vi "Gather Input.vi"(4 "Shifter":T1, 7 "Gamepad":T1, 8 "Joystick Right":T1, 11 "Joystick Left":T1) -> ()   [LabVIEW 2016]
uses:
  <vilib>/Rock Robotics/WPI/Joystick/WPI_JoystickDevRef.ctl
  <vilib>/Rock Robotics/WPI/Joystick/WPI_JoystickDeviceEnum.ctl
  Joystick Values.vi
panel:
  in  "Gamepad 2":T1
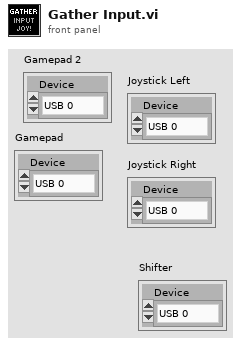
[diagram p1: front panel]
types:
  T1 = typedef "WPI_JoystickDevRef.ctl" = cluster{"Device":T2}
  T2 = typedef "WPI_JoystickDeviceEnum.ctl" = enum16{"USB 0", "USB 1", "USB 2", "USB 3", "USB 4", "USB 5"}
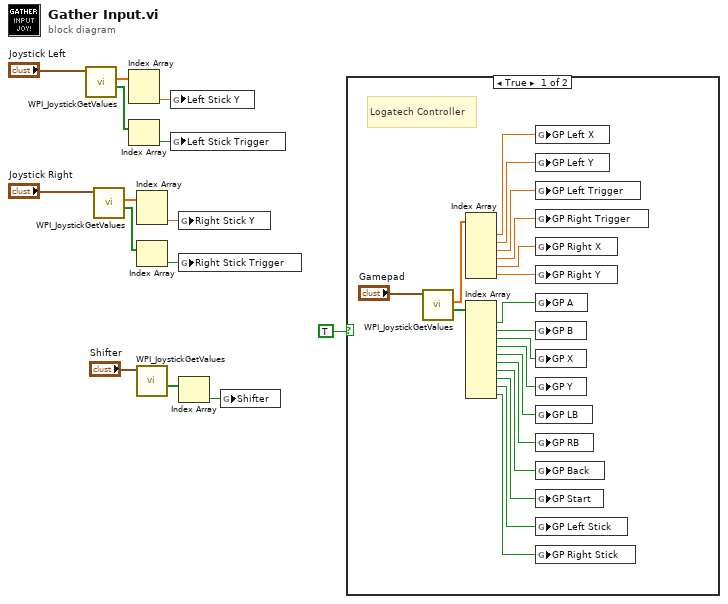
[diagram p0: block diagram]
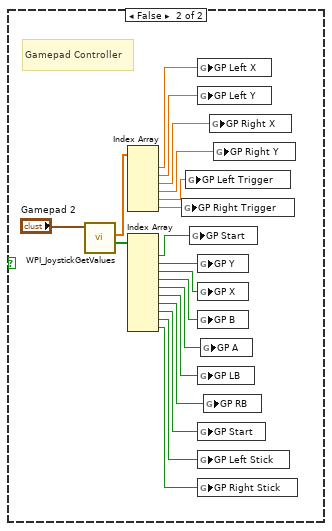
[diagram p2: hidden frame]
diagram:
  n1 = call <vilib>:"WPI_JoystickGetValues.vi"("JoystickDevRef"="Joystick Left") -> ("Buttons"=w6:bool[], "Axes"=w5:dbl[])  [unwired: 6 in, 3 out]
  n2 = call <vilib>:"WPI_JoystickGetValues.vi"("JoystickDevRef"="Joystick Right") -> ("Buttons"=w12:bool[], "Axes"=w10:dbl[])  [unwired: 6 in, 3 out]
  n3 = Index Array(array=w5) -> (element #2=w7:dbl)  [unwired: 2 in, 1 out]
  n4 = Index Array(array=w6) -> (element=w8:bool)  [unwired: 1 in]
  n5 = Index Array(array=w10) -> (element #2=w9:dbl)  [unwired: 2 in, 1 out]
  n6 = Index Array(array=w12) -> (element=w11:bool)  [unwired: 1 in]
  n7 = call <vilib>:"WPI_JoystickGetValues.vi"("JoystickDevRef"="Shifter") -> ("Buttons"=w3:bool[])  [unwired: 6 in, 4 out]
  n8 = global write "Joystick Values.vi" "Left Stick Y"(w7) -> ()
  n9 = global write "Joystick Values.vi" "Left Stick Trigger"(w8) -> ()
  n10 = global write "Joystick Values.vi" "Right Stick Y"(w9) -> ()
  n11 = global write "Joystick Values.vi" "Right Stick Trigger"(w11) -> ()
  n12 = Index Array(array=w3) -> (element=w2:bool)  [unwired: 1 in]
  n13 = global write "Joystick Values.vi" "Shifter"(w2) -> ()
  n14 = case shown="True" TRUE {
    frame True {
      # "Logatech Controller"
      n15 = call <vilib>:"WPI_JoystickGetValues.vi"("JoystickDevRef"="Gamepad") -> ("Buttons"=w32:bool[], "Axes"=w20:dbl[])  [unwired: 6 in, 3 out]
      n16 = Index Array(array=w20) -> (element #1=w21:dbl, element #2=w19:dbl, element #3=w16:dbl, element #4=w15:dbl, element #5=w18:dbl, element #6=w17:dbl)  [unwired: 6 in]
      n17 = Index Array(array=w32) -> (element #1=w31:bool, element #2=w30:bool, element #3=w29:bool, element #4=w28:bool, element #5=w27:bool, element #6=w26:bool, element #7=w25:bool, element #8=w24:bool, element #9=w23:bool, element #10=w22:bool)  [unwired: 10 in]
      n18 = global write "Joystick Values.vi" "GP Left X"(w21) -> ()
      n19 = global write "Joystick Values.vi" "GP Left Y"(w19) -> ()
      n20 = global write "Joystick Values.vi" "GP Left Trigger"(w16) -> ()
      n21 = global write "Joystick Values.vi" "GP Right Trigger"(w15) -> ()
      n22 = global write "Joystick Values.vi" "GP Right X"(w18) -> ()
      n23 = global write "Joystick Values.vi" "GP Right Y"(w17) -> ()
      n24 = global write "Joystick Values.vi" "GP A"(w31) -> ()
      n25 = global write "Joystick Values.vi" "GP B"(w30) -> ()
      n26 = global write "Joystick Values.vi" "GP X"(w29) -> ()
      n27 = global write "Joystick Values.vi" "GP Y"(w28) -> ()
      n28 = global write "Joystick Values.vi" "GP LB"(w27) -> ()
      n29 = global write "Joystick Values.vi" "GP RB"(w26) -> ()
      n30 = global write "Joystick Values.vi" "GP Back"(w25) -> ()
      n31 = global write "Joystick Values.vi" "GP Start"(w24) -> ()
      n32 = global write "Joystick Values.vi" "GP Left Stick"(w23) -> ()
      n33 = global write "Joystick Values.vi" "GP Right Stick"(w22) -> ()
    }
    frame False {
      # "Gamepad Controller"
      n34 = call <vilib>:"WPI_JoystickGetValues.vi"("JoystickDevRef"="Gamepad 2") -> ("Buttons"=w51:bool[], "Axes"=w39:dbl[])  [unwired: 6 in, 3 out]
      n35 = Index Array(array=w39) -> (element #1=w40:dbl, element #2=w38:dbl, element #3=w35:dbl, element #4=w34:dbl, element #5=w37:dbl, element #6=w36:dbl)  [unwired: 6 in]
      n36 = Index Array(array=w51) -> (element #1=w50:bool, element #2=w49:bool, element #3=w48:bool, element #4=w47:bool, element #5=w46:bool, element #6=w45:bool, element #7=w44:bool, element #8=w43:bool, element #9=w42:bool, element #10=w41:bool)  [unwired: 10 in]
      n37 = global write "Joystick Values.vi" "GP Right Trigger"(w36) -> ()
      n38 = global write "Joystick Values.vi" "GP Left Trigger"(w37) -> ()
      n39 = global write "Joystick Values.vi" "GP Start"(w50) -> ()
      n40 = global write "Joystick Values.vi" "GP Left X"(w40) -> ()
      n41 = global write "Joystick Values.vi" "GP Left Y"(w38) -> ()
      n42 = global write "Joystick Values.vi" "GP Y"(w49) -> ()
      n43 = global write "Joystick Values.vi" "GP X"(w48) -> ()
      n44 = global write "Joystick Values.vi" "GP B"(w47) -> ()
      n45 = global write "Joystick Values.vi" "GP LB"(w45) -> ()
      n46 = global write "Joystick Values.vi" "GP Start"(w43) -> ()
      n47 = global write "Joystick Values.vi" "GP Left Stick"(w42) -> ()
      n48 = global write "Joystick Values.vi" "GP Right Stick"(w41) -> ()
      n49 = global write "Joystick Values.vi" "GP A"(w46) -> ()
      n50 = global write "Joystick Values.vi" "GP RB"(w44) -> ()
      n51 = global write "Joystick Values.vi" "GP Right X"(w35) -> ()
      n52 = global write "Joystick Values.vi" "GP Right Y"(w34) -> ()
    }
  }
